vi "HW_QX_Choose Connect Device UI.vi"(8 "error in":errorcluster) -> (0 "error out":errorcluster, 3 "QX Dev":T2)   [LabVIEW 2016]
doc: "搜索系统中网络设备信息\n通过勾选确定需要连接的设备"
uses:
  <vilib>/Utility/error.llb/DialogType.ctl
  Ctrls/Wizard_Cancel Button.ctl
  Ctrls/Wizard_OK Button.ctl
  Ctrls/Wizard_Scan Button.ctl
  QX Module Info.ctl
panel:
  in  "TempVariable":T3
  out "Error Report":string
  out "Current State":string
  in  "Cancel":T4
  in  "OK":T5
  in  "Scan":T6
  out "DevList":i32(listbox) caption="选择连接设备..."
  # "/* -------- Notes for All Users -------- */\nRecommand : \n[1].Display Setting Resolution -> 1440x900\n[2].Read Arch Notes First.\n[3].Make A Call When You Are In Trouble.\n\nTeam Members:\nPansino Soft,Pansino SDMA\n\nCopyright@2013 Pansino.Beijing\n\nVersion Number: 2013"
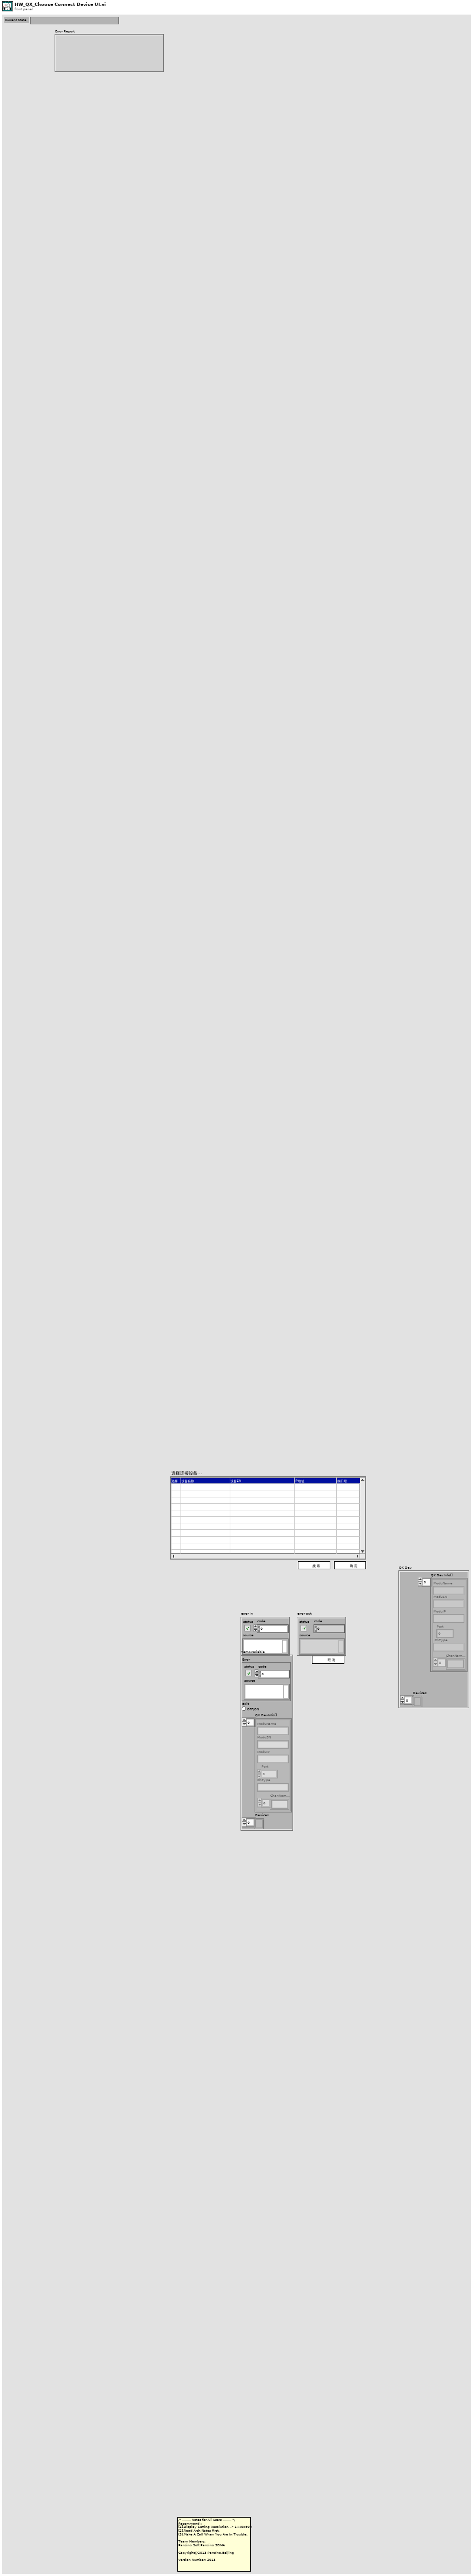
[diagram p1: front panel]
types:
  T1 = typedef "QX Module Info.ctl" = cluster{"ModuName":string, "ModuSN":string, "ModuIP":string, "Port":i32, "ChType":string, "ChanNames[]":string[]}
  T2 = cluster{"QX DevInfo[]":T1[], "Devices":refnum<k24>[]}
  T3 = cluster{"Error":errorcluster, "Exit":bool, "QX DevInfo[]":T1[], "Devices":refnum<k24>[]}
  T4 = typedef "Wizard_Cancel Button.ctl" = bool
  T5 = typedef "Wizard_OK Button.ctl" = bool
  T6 = typedef "Wizard_Scan Button.ctl" = bool
  T7 = enum32{"Invalid", "Standard", "Closed", "Hidden", "Minimized", "Maximized"}
  T8 = typedef "LVPoint32TypeDef.ctl" = cluster{"Horizontal":i32, "Vertical":i32}
  T9 = typedef "LVRowAndColumnTypeDef.ctl" = cluster{"Row":i32, "Column":i32}
  T10 = typedef "DialogType.ctl" = u16
  T11 = cluster{"ParaFolder":path, "SysCfg":path, "CHdef":path, "ModCfg":path, "DT Folder":path, "ErrorLog":path, "HBMDriverlicense":path}
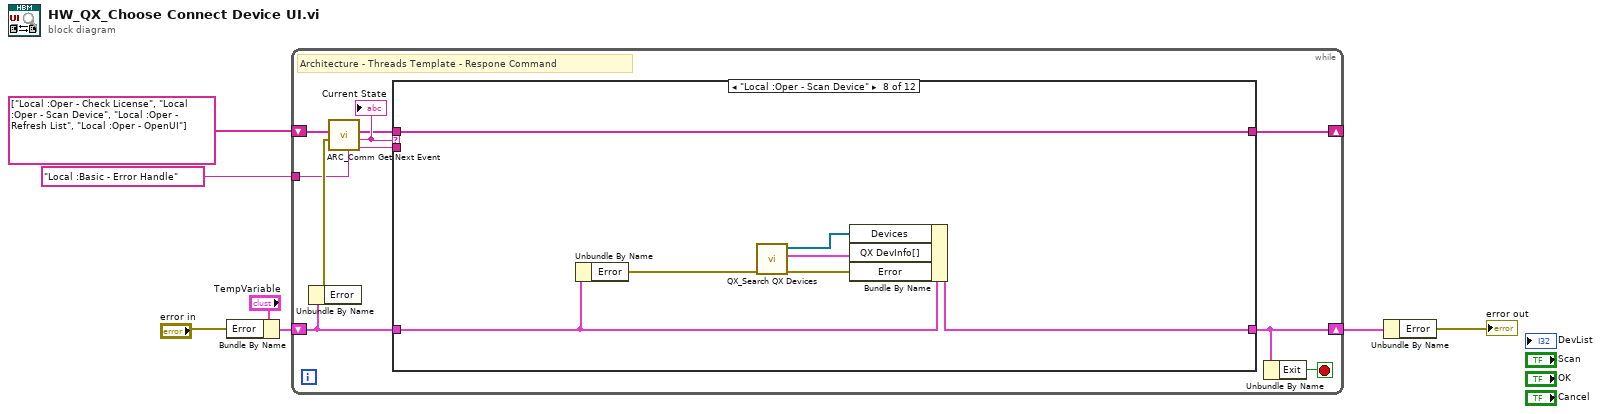
[diagram p0: block diagram]
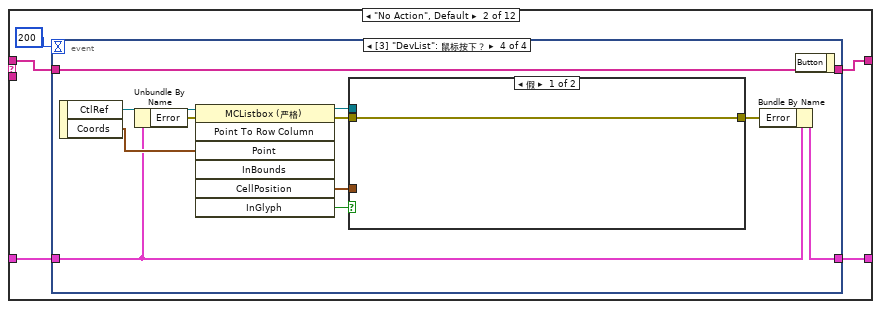
[diagram p3: hidden frame]
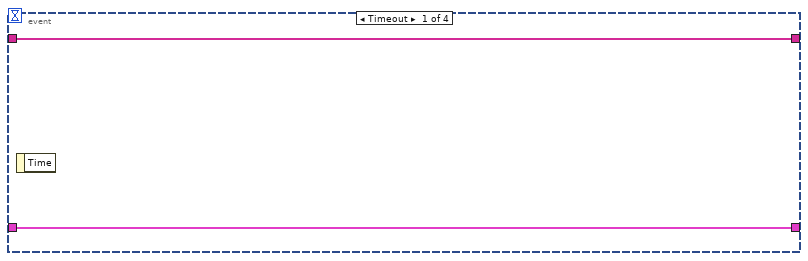
[diagram p4: hidden frame]
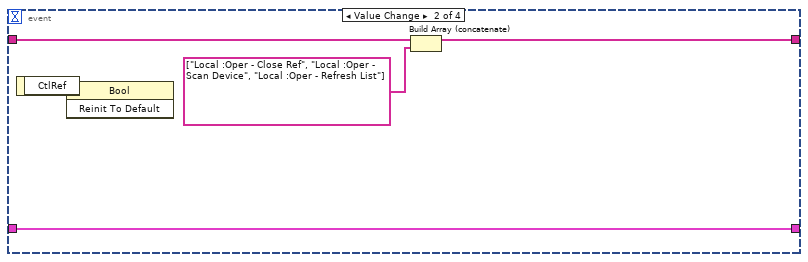
[diagram p5: hidden frame]
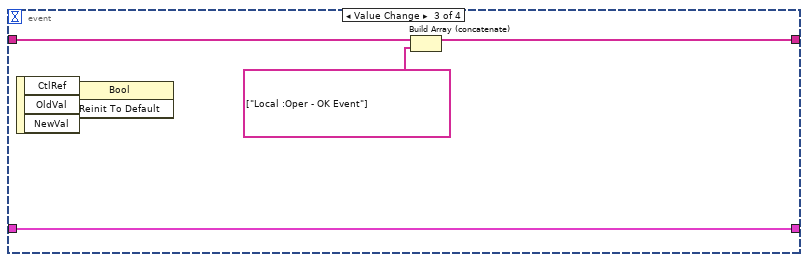
[diagram p6: hidden frame]
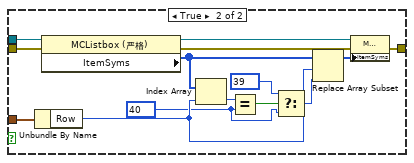
[diagram p7: hidden frame]
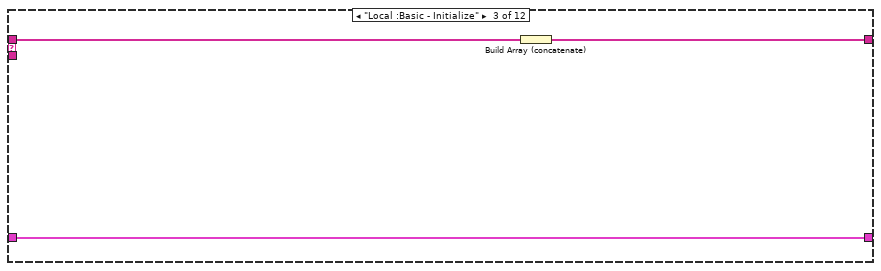
[diagram p8: hidden frame]
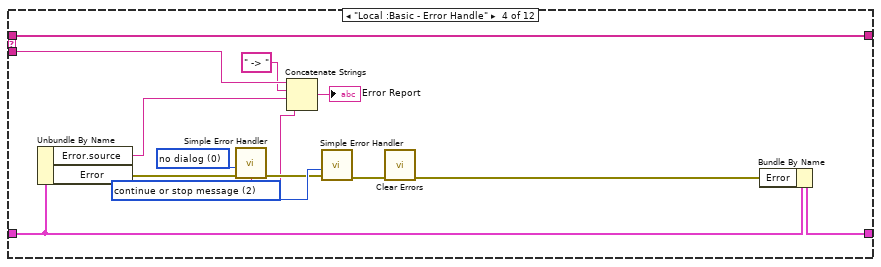
[diagram p9: hidden frame]
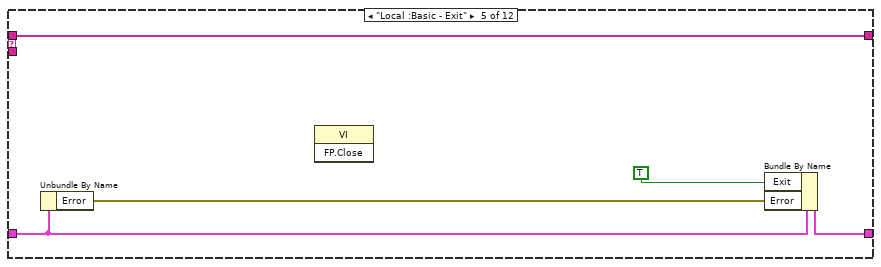
[diagram p10: hidden frame]
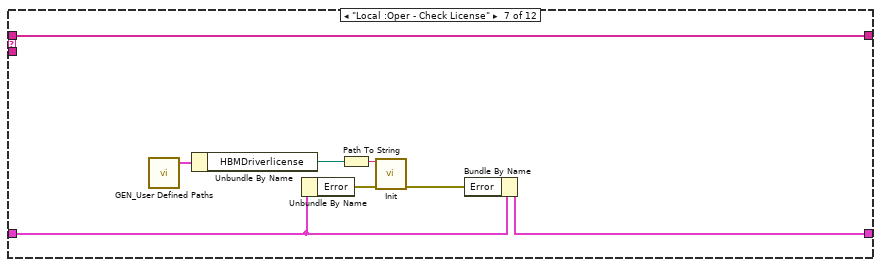
[diagram p12: hidden frame]
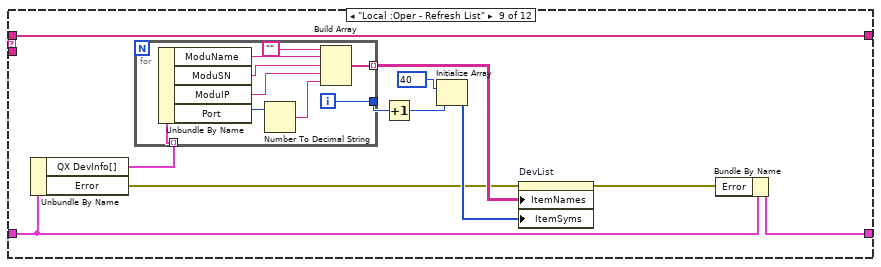
[diagram p13: hidden frame]
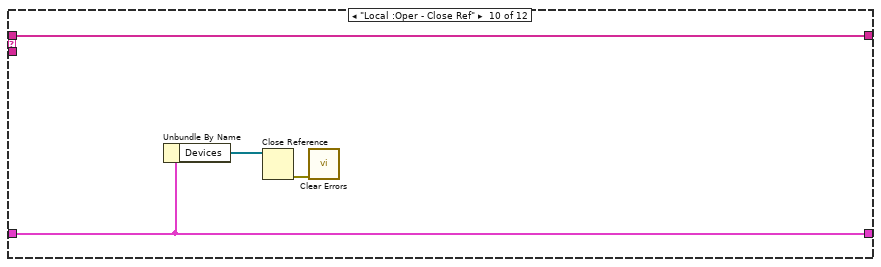
[diagram p14: hidden frame]
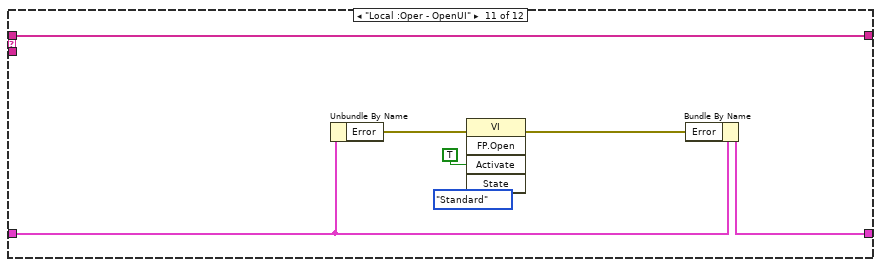
[diagram p15: hidden frame]
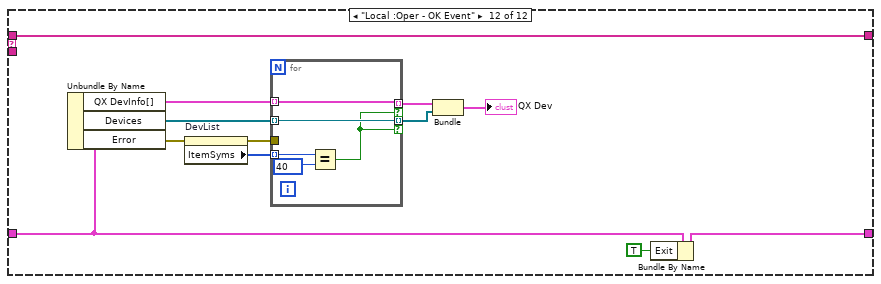
[diagram p16: hidden frame]
diagram:
  n1 = Bundle By Name(cluster="TempVariable", "Error"="error in") -> (w3:T3)
  n2 = while {
    shift-right: [w11] -> w7
    shift-left: w3 -> [w13]
    shift-right: [w14] -> _
    shift-left: string[] ["Local :Oper - Check License", "Local :Oper - Scan Device", "Local :Oper - Refresh List", "Local :Oper - OpenUI"] ("appended array") -> [w17]
    tunnel: "Local :Basic - Error Handle" ("Error Handle") -> [w9]
    stop <- w10 stop-if-true
    # "Architecture - Threads Template - Respone Command"
    n3 = Unbundle By Name(w13) -> ("Error"=w12:errorcluster)
    n4 = call "ARC_Comm Get Next Event.vi"("Error Handle"=w9, "error in (no error)"=w12, "event queue in"=w17) -> ("prev event"=w8:string, "next event"=w16:string, "event queue out"=w15:string[])  [unwired: 3 in]
    "Current State" <- w16
    n5 = case shown="\"Local :Oper - Scan Device\"" w16 {
      tunnel: w13 -> [w18 w21 w64 w77 w81 w85 w90 w100 w106 w124 w129 w143]
      tunnel: w15 -> [w19 w24 w65 w79 w84 w86 w94 w101 w112 w125 w132 w144]
      tunnel: [w19 w23 w63 w79 w84 w86 w94 w101 w112 w125 w132 w144] -> w14
      tunnel: [w18 w20 w64 w78 w82 w85 w88 w99 w103 w124 w127 w134] -> w11
      tunnel: w8 -> [_ _ _ w70 _ _ _ _ _ _ _ _]
      frame "----------Core Status----------" {
      }
      frame "No Action", Default {
        n6 = event shown="[3] \"DevList\": 鼠标按下？" {
          selector: _ -> [_ _ _ _]
          dyn-events: _ -> [_ _ _ _]
          timeout: 200 -> [_ _ _ _]
          tunnel: w24 -> [w26 w31 w36 w47]
          tunnel: [w26 w28 w33 w47] -> w23
          tunnel: w21 -> [w25 w30 w35 w44]
          tunnel: [w25 w30 w35 w38] -> w20
          event Timeout {
            n7 = event-data() -> ()  [unwired: 1 in, 1 out]
          }
          event Value Change {
            n8 = event-data() -> ("CtlRef"=w29:refnum<vi>)  [unwired: 1 in]
            n9 = invoke class="Bool" method="Reinit To Default"(reference=w29) -> ()  [unwired: 2 in, 3 out]
            n10 = Build Array (concatenate)(w31, string[] ["Local :Oper - Close Ref", "Local :Oper - Scan Device", "Local :Oper - Refresh List"] ("appended array")) -> (w28:string[])
          }
          event Value Change {
            n11 = event-data() -> ("CtlRef"=w34:refnum<vi>)  [unwired: 1 in, 2 out]
            n12 = invoke class="Bool" method="Reinit To Default"(reference=w34) -> ()  [unwired: 2 in, 3 out]
            n13 = Build Array (concatenate)(w36, string[] ["Local :Oper - OK Event"] ("appended array")) -> (w33:string[])
          }
          event "DevList": Mouse Down? {
            n14 = event-data() -> ("CtlRef"=w46:refnum<vi>, "Coords"=w45:T8)  [unwired: 1 in]
            n15 = Unbundle By Name(w44) -> ("Error"=w43:errorcluster)
            n16 = invoke class="MCListbox (严格)" method="Point To Row Column"(reference=w46, error in=w43, "Point"=w45) -> (reference out=w41:refnum<vi>, error out=w40:errorcluster, "CellPosition"=w39:T9, "InGlyph"=w42:bool)  [unwired: 4 in, 3 out]
            n17 = case shown="假" w42 {
              tunnel: w41 -> [_ w62]
              tunnel: w40 -> [w48 w61]
              tunnel: w39 -> [_ w60]
              tunnel: [w48 w49] -> w37
              frame False {
              }
              frame True {
                w54 = 40
                n18 = Unbundle By Name(w60) -> ("Row"=w58:i32)
                n19 = property class="MCListbox (严格)"(reference=w62, error in=w61) -> (reference out=w51:refnum<vi>, error out=w50:errorcluster, "ItemSyms"=w57:i32[])
                n20 = Index Array(array=w57, index=w58) -> (element=w59:i32)
                n21 = Equal?(x=w59, y=w54) -> (x = y?=w56:bool)
                n22 = Select(t=39, s=w56, f=w54) -> (s? t:f=w53:i32)
                n23 = Replace Array Subset(array=w57, new element=w53, index=w58) -> (w52:i32[])
                n24 = property class="MCListbox (strict)"(reference=w51, error in=w50, "ItemSyms"=w52) -> (error out=w49:errorcluster)  [unwired: 1 out]
              }
            }
            n25 = Bundle By Name(cluster=w44, "Error"=w37) -> (w38:T3)
            n26 = event-data() -> ()  [unwired: 2 in, 1 out]
          }
        }
      }
      frame "Local :Basic - Initialize" {
        n27 = Build Array (concatenate)(w65) -> (w63:string[])
      }
      frame "Local :Basic - Error Handle" {
        w71 = T10 0 items=["no dialog", "OK message", "continue or stop message", "OK message + warnings", "continue/stop + warnings"] ("type of dialog (OK msg:1)")
        w74 = T10 2 items=["no dialog", "OK message", "continue or stop message", "OK message + warnings", "continue/stop + warnings"] ("type of dialog (OK msg:1)")
        n28 = Unbundle By Name(w77) -> ("Error.source"=w66:string, "Error"=w73:errorcluster)
        n29 = call <vilib>:"Simple Error Handler.vi"("type of dialog (OK msg:1)"=w71, "error in (no error)"=w73) -> ("error out"=w72:errorcluster, "message"=w68:string)  [unwired: 3 in, 3 out]
        n30 = Concatenate Strings(w70, " -> " ("字符串"), w66, w68) -> (→"Error Report":string)
        n31 = call <vilib>:"Simple Error Handler.vi"("type of dialog (OK msg:1)"=w74, "error in (no error)"=w72) -> ("error out"=w76:errorcluster)  [unwired: 3 in, 4 out]
        n32 = call <vilib>:"Clear Errors.vi"("error in (no error)"=w76) -> ("error out"=w75:errorcluster)  [unwired: 5 in, 1 out]
        n33 = Bundle By Name(cluster=w77, "Error"=w75) -> (w78:T3)
      }
      frame "Local :Basic - Exit" {
        n34 = Unbundle By Name(w81) -> ("Error"=w83:errorcluster)
        n35 = invoke class="VI" method="FP.Close"() -> ()  [unwired: 3 in, 3 out]
        n36 = Bundle By Name(cluster=w81, "Exit"=TRUE, "Error"=w83) -> (w82:T3)
      }
      frame "---------------------------------" {
      }
      frame "Local :Oper - Check License" {
        n37 = call "GEN_User Defined Paths.vi"() -> ("UserDefinedPath"=w93:T11)  [unwired: 11 in]
        n38 = Unbundle By Name(w93) -> ("HBMDriverlicense"=w92:path)
        n39 = Unbundle By Name(w90) -> ("Error"=w89:errorcluster)
        n40 = Path To String(path=w92) -> (string=w91:string)
        n41 = call "Init.vi"("LicenseFileName"=w91, "Error in"=w89) -> ("Error out"=w87:errorcluster)  [unwired: 6 in, 2 out]
        n42 = Bundle By Name(cluster=w90, "Error"=w87) -> (w88:T3)
      }
      frame "Local :Oper - Scan Device" {
        n43 = Unbundle By Name(w100) -> ("Error"=w95:errorcluster)
        n44 = call "QX_Search QX Devices.vi"("error in"=w95) -> ("error out"=w98:errorcluster, "QX DevInfo"=w97:T1[], "Devices"=w96:refnum<k24>[])  [unwired: 8 in]
        n45 = Bundle By Name(cluster=w100, "Devices"=w96, "QX DevInfo[]"=w97, "Error"=w98) -> (w99:T3)
      }
      frame "Local :Oper - Refresh List" {
        n46 = Unbundle By Name(w106) -> ("QX DevInfo[]"=w105:T1[], "Error"=w104:errorcluster)
        n47 = for {
          tunnel: w105 -> [w121] mode=indexing
          tunnel: [w115] -> w111 mode=indexing
          tunnel: [w113] -> w110
          i -> [w113]
          n48 = Unbundle By Name(w121) -> ("ModuName"=w119:string, "ModuSN"=w118:string, "ModuIP"=w117:string, "Port"=w120:i32)
          n49 = Number To Decimal String(number=w120) -> (decimal integer string=w116:string)  [unwired: 1 in]
          n50 = Build Array("", w119, w118, w117, w116) -> (w115:string[])
        }
        n51 = Increment(x=w110) -> (x+1=w109:i32)
        n52 = Initialize Array(40, w109) -> (w107:i32[])
        n53 = property on="DevList" class="MCListbox (严格)"(error in=w104, "ItemNames"=w111, "ItemSyms"=w107) -> (error out=w102:errorcluster)  [unwired: 1 in, 1 out]
        n54 = Bundle By Name(cluster=w106, "Error"=w102) -> (w103:T3)
      }
      frame "Local :Oper - Close Ref" {
        n55 = Unbundle By Name(w124) -> ("Devices"=w123:refnum<k24>[])
        n56 = Close Reference(reference=w123) -> (error out=w122:errorcluster)  [unwired: 1 in]
        n57 = call <vilib>:"Clear Errors.vi"("error in (no error)"=w122) -> ()  [unwired: 5 in, 2 out]
      }
      frame "Local :Oper - OpenUI" {
        n58 = Unbundle By Name(w129) -> ("Error"=w128:errorcluster)
        n59 = invoke class="VI" method="FP.Open"(error in=w128, "Activate"=TRUE ("Activate?"), "State"=T7."Standard") -> (error out=w126:errorcluster)  [unwired: 2 in, 4 out]
        n60 = Bundle By Name(cluster=w129, "Error"=w126) -> (w127:T3)
      }
      frame "Local :Oper - OK Event" {
        n61 = Unbundle By Name(w143) -> ("QX DevInfo[]"=w141:T1[], "Devices"=w140:refnum<k24>[], "Error"=w142:errorcluster)
        n62 = property on="DevList" class="MCListbox (严格)"(error in=w142) -> (error out=w139:errorcluster, "ItemSyms"=w138:i32[])  [unwired: 1 in, 1 out]
        n63 = for {
          tunnel: w141 -> [w147] mode=indexing
          tunnel: w140 -> [w146] mode=indexing
          tunnel: w139 -> [_]
          tunnel: w138 -> [w149] mode=indexing
          tunnel: [w147] -> w137 mode=indexing if=w145
          tunnel: [w146] -> w136 mode=indexing if=w145
          n64 = Equal?(x=w149, y=40) -> (x = y?=w145:bool)
        }
        n65 = Bundle(w137, w136) -> (→"QX Dev":cluster{T1[], refnum<k24>[]})  [unwired: 1 in]
        n66 = Bundle By Name(cluster=w143, "Exit"=TRUE) -> (w134:T3)
      }
    }
    n67 = Unbundle By Name(w11) -> ("Exit"=w10:bool)
  }
  n68 = Unbundle By Name(w7) -> ("Error"=→"error out":errorcluster)
